vi "1.0.1_Set_SKU_Config.vi"(8 "error in (no error)":errorcluster, 10 "?":T1, 11 "Message Queue out":T2) -> (0 "error out":errorcluster, 1 "Flow":string, 2 "Data":T1, 3 "Message Queue Out":T2)   [LabVIEW 2017]
uses:
  DIPC 692 Daemon API/typdef/destination.ctl
  Depends/AMC/subVIs/TypeDefs/amc_Message Queue.ctl
  Depends/AMC/subVIs/TypeDefs/amc_Message.ctl
  Depends/Tools/Keyed Array/Tools_KeyedArray KeyedArray.ctl
  Ctrls/Data.ctl
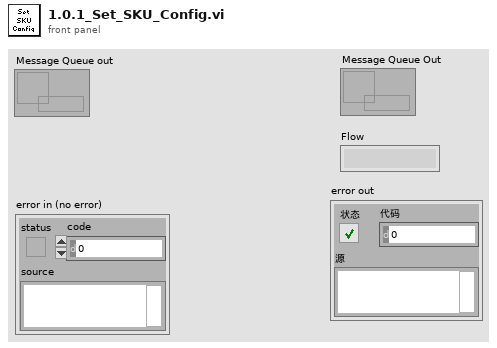
[diagram p1: front panel]
types:
  T1 = typedef "Data.ctl" = cluster{"SN":string, "Start Time":timestamp, "Step Time":timestamp, "Count":cluster{"Total":i32, "OK":i32, "NG":i32, "Yield":dbl}, "Table":string[][], "daemon reference":refnum<k5>, "CT":dbl, "Config":string[][], "Initialisation":cluster{"Set_SKU_Config_With_LMT":string, "FCT_timestamp":string, "sw_version_before":string, "hardware_serial":string, "Backup_DDM_NVM":string, "Flash_SW_follow_SKU":string, "sw_version_after":string, "Set_SKU_Config_base_on_variant":string, "UUT_Ready_Status":string, "Set_DDM_to_EOL_Mode":string, "DDM_Parameter":dbl[], "DDM_Parameter_status":bool[], "Get_Tester_Parameter":dbl[], "Get_Tester_Parameter_status":bool[], "Cal_Tester_Parameter":dbl[], "Cal_Tester_Parameter_status":bool[], "sw_version_before_status":bool, "sw_version_after_status":bool, "Reflashing_Flash_SW_follow_SKU":string, "Set_SKU_Config_With_LMT_status":bool, "FCT_timestamp_status":bool}, "BEMF_Calibration":cluster{"Read_ambient_temperature":dbl, "Set_ambient_temperature_to_DDM":string, "Save_Calibration":string, "Calibration_Vaule":dbl[], "Calibration_Start_Calibration":string, "Calibration_Vaule _B":dbl[], "Calibration_Vaule_status":bool[], "Calibration_Vaule_B_status":bool[]}, "ECO":cluster{"Reset_Power_tune_vaule_to_zero":string, "ECO_Motor_On_with_power_mode":string, "DDM_Parameter":dbl[], "DDM_Parameter_status":bool[], "Get_Tester_Parameter":dbl[], "Get_Tester_Parameter_status":bool[], "Cal_Tester_Parameter":dbl[], "Cal_Tester_Parameter_status":bool[], "DDM_Parameter_after_power_tune":dbl[], "Get_Tester_Parameter_after_power_tune":dbl[], "Cal_Tester_Parameter_after_power_tune":dbl[], "Cal_Tester_Parameter_after_power_tune_status":bool[], "Delta_P":dbl, "ECO_Power_Tune_Set_Delta_Power_tune_value_to_DDM":string, "ECO_Power_Tune_Motor_On_with_power_mode":string, "Reset_BEMF_FISF_calibration":string}, "BOOST":cluster{"DDM_Parameter":dbl[], "DDM_Parameter_status":bool[], "Get_Tester_Parameter":dbl[], "Get_Tester_Parameter_status":bool[], "Cal_Tester_Parameter":dbl[], "Cal_Tester_Parameter_status":bool[], "DDM_Parameter_after_power_tune":dbl[], "Get_Tester_Parameter_after_power_tune":dbl[], "Cal_Tester_Parameter_after_power_tune":dbl[], "Cal_Tester_Parameter_after_power_tune_status":bool[], "airwatts_am_off":dbl, "AW_Delta_(AM_on_and_off)":dbl, "AW_Delta_(AM_on_and_off)_Status":bool, "Delta_P":dbl, "BOOST_Motor_On_with_power_mode":string, "BOOST_Air_Muscle_Check_Turn_off_air_muscle":string, "BOOST_Power_Tune_Set_Delta_Power_tune_value_to_DDM":string, "BOOST_Power_Tune_Motor_On_with_power_mode":string, "BOOST_Stop_motor":string, "BOOST_Save_Calibration":string, "BOOST_Get_AW_Calibration_value":string}, "MAX":cluster{"Max_Motor_On_with_power_mode":string, "Average_Tmag_Data":cluster{"LSI Delta in degC":dbl, "FISF Delta in degc":dbl, "LSI Tmag in degC":dbl, "Fisf Tmag in degC":dbl, "IIR Tmag in degC":dbl}, "DDM_Parameter":dbl[], "DDM_Parameter_status":bool[], "Get_Tester_Parameter":dbl[], "Get_Tester_Parameter_status":bool[], "Cal_Tester_Parameter":dbl[], "BEMF_Finetune":cluster{"eol_bemf_mp_cold_coef_c":dbl, "eol_cold_bemf_fisf_offset":dbl}, "AW_Tune":cluster{"delta_P1":dbl, "delta_P_Setting":dbl}, "DDM_Parameter_after_Airwatts_Tune":dbl[], "Get_Tester_Parameter_after_Airwatts_Tune":dbl[], "Cal_Tester_Parameter_after_Airwatts_Tune":dbl[], "AW_after_Airwatts_Tune":bool, "DDM_Parameter_after_Airwatts_Finetune":dbl[], "Get_Tester_Parameter_after_Airwatts_Finetune":dbl[], "Cal_Tester_Parameter_after_Airwatts_Finetune":dbl[], "AW_after_Airwatts_Finetune":bool, "AW_Finetune":cluster{"delta_P2":dbl, "delta_P_Setting":dbl}, "Delta_Tmag_after_tune":cluster{"LSI Delta in degC":dbl, "FISF Delta in degc":dbl, "LSI Tmag in degC":dbl, "Fisf Tmag in degC":dbl, "IIR Tmag in degC":dbl}, "Hot Bemf in mV":dbl, "DDM_Pressure":dbl, "Delta_Pressure":dbl, " Cold Bemf in mV":dbl, " delta Bemf":dbl, " delta p":dbl, "Delta_Pressure_status":bool, " delta Bemf_status":bool, "LSI Delta in degC_status":bool, "FISF Delta in degc_status":bool, "Motor_On_with_power_mode_after_Airwatts_Tune":string, "Airwatts_Finetune_Motor_On_with_power_mode":string, "Airwatts_Finetune_Stop_motor":string, "Max_check_derate_status":string, "Max_Stop_motor":string, "Max_Save_Calibration":string, "AW":bool, "Max_check_derate_status_status":bool, "Average_All_data":dbl[][], "Average_Tmag_Data_status":bool[], "Average_Tmag_Data_after_tune_status":bool[]}, "Task_Detect_Calib":cluster{"LL":cluster{"DDM_Parameter":dbl[], "DDM_Parameter_status":bool[], "Get_Tester_Parameter":dbl[], "Get_Tester_Parameter_status":bool[], "Set_task_detect_A":dbl, "LL_Motor_On":string}, "HL":cluster{"DDM_Parameter":dbl[], "DDM_Parameter_status":bool[], "Get_Tester_Parameter":dbl[], "Get_Tester_Parameter_status":bool[], "Set_task_detect_B":dbl, "HL_Motor_On":string, "HL_Motor_Stop":string}, "LH":cluster{"DDM_Parameter":dbl[], "DDM_Parameter_status":bool[], "Get_Tester_Parameter":dbl[], "Get_Tester_Parameter_status":bool[], "Set_task_detect_C":dbl, "LH_Motor_On":string}, "HH":cluster{"DDM_Parameter":dbl[], "DDM_Parameter_status":bool[], "Get_Tester_Parameter":dbl[], "Get_Tester_Parameter_status":bool[], "Set_task_detect_D":dbl, "HH_Motor_On":string, "HH_Set_calibration_eol_inlet_blockage":string, "HH_Motor_Stop":string, "HH_Save_calibration":string}, "Get_eol_inlet_blockage_E":dbl, "Calib_vaule":cluster{"Get_task_detect_LL":dbl, "Get_task_detect_HL":dbl, "Get_task_detect_LH":dbl, "Get_task_detect_HH":dbl, "eol_inlet_blockage":dbl}, "Reset_all_task_detect_calibration_parameter":string, "calibrated temp":dbl, "Set ambient temperature to DDM":string, "Set ambient temperature to DDM after task detect":string, "Inlet_Blockage_Calibration":cluster{"DDM_Parameter":dbl[], "DDM_Parameter_status":bool[], "Get_Tester_Parameter":dbl[], "Get_Tester_Parameter_status":bool[], "Inlet_Blockage_Calibration_Motor_On":string, "Calibrate Inlet Blockage":string}}, "good":cluster{"Write_Product_TS":cluster{"TIMESTAMP":i64, "RIG_ID":i64, "PASSMARK_ID":i64, "PASSMARK_REV":i64}, "Read_Product_TS":cluster{"TIMESTAMP":i64, "RIG_ID":i64, "PASSMARK_ID":i64, "PASSMARK_REV":i64}, "Good_Clear_NVM_Error":string, "Good_Set_DDM_to_Product_mode":string, "Good_Write_Product_Timestamp":string, "Good_Read_Product_Timestamp":string, "Good_Backup_DDM_NVM":string, "Good_Set_Secuity_Bit":string, "Good_Set_Calibration_Lock":string, "Good_Check_Secuity_Bit":string, "Good_Check_Secuity_Bit_Stauts":bool}, "Buyoff":cluster{"bit_status":string, "cold_bemf_temp":dbl, "BEMF_Calib_data":dbl[], "AW_Tune_Calib_data":dbl[], "task_Calib_data":dbl[], "Read_Product_TS":cluster{"TIMESTAMP":i64, "RIG_ID":i64, "PASSMARK_ID":i64, "PASSMARK_REV":i64}, "lock_status":string, "Functionality_Buyoff_Get_Product_Timestamp":string}, "UUT_Type":enum16{"692", "692B", "692D"}, "NG":cluster{"NG_Read_Error":string, "NG_Change_to_FCT_mode":string, "NG_Backup_DDM_NVM":string}, "OK/NG":bool}
  T2 = typedef "amc_Message Queue.ctl" = refnum<queue>
  T3 = typedef "HD Config.ctl" = cluster{" PC":cluster{"PC Address":u8[], "PC Port":i32}, "FCO":cluster{"COM":refnum<visa-resource-name>, "Baudrate":u32}, "DC Power ":cluster{"COM":refnum<visa-resource-name>, "Baudrate":u32}, "PW3336":cluster{"COM":refnum<visa-resource-name>, "Baudrate":u32}, "Lefoo":cluster{"COM":refnum<visa-resource-name>, "Baudrate":u32}, "AI Model":cluster{"COM":refnum<visa-resource-name>, "Baudrate":u32}, "DIPC":cluster{"COM":refnum<visa-resource-name>}, "Daemon":cluster{"IP Address":string, "Port":u16}, "Motor":cluster{"COM":refnum<visa-resource-name>, "Baudrate":u32}}
  T4 = typedef "destination.ctl" = string
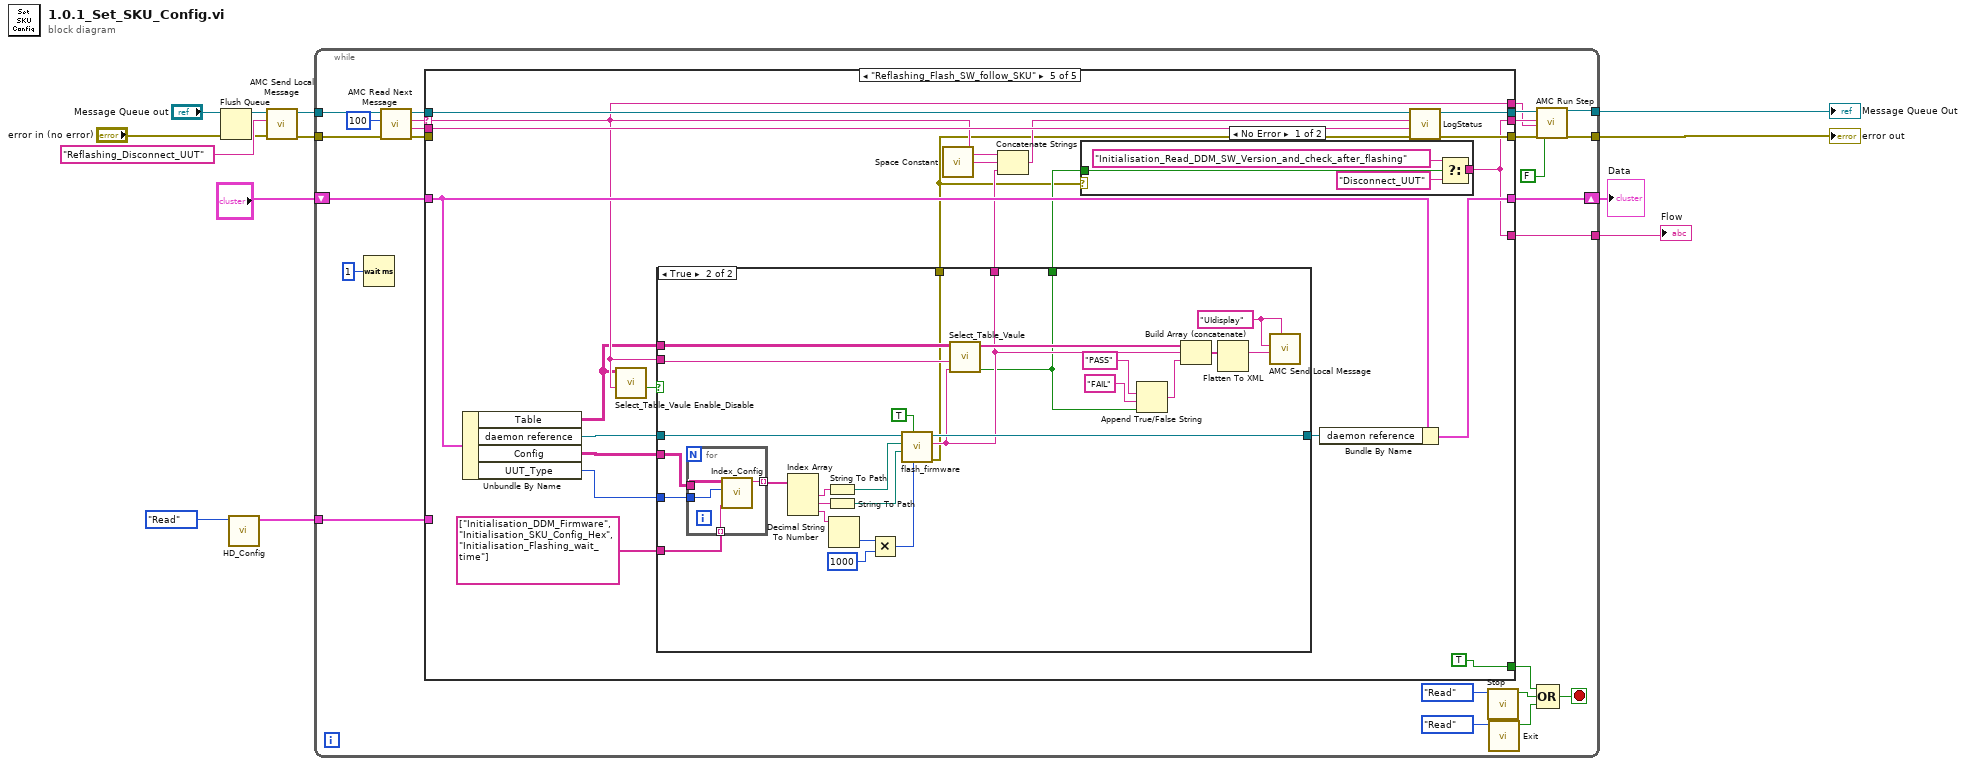
[diagram p0: block diagram]
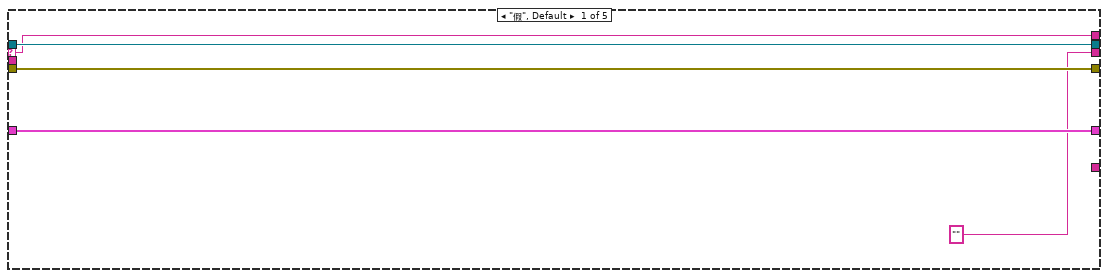
[diagram p2: hidden frame]
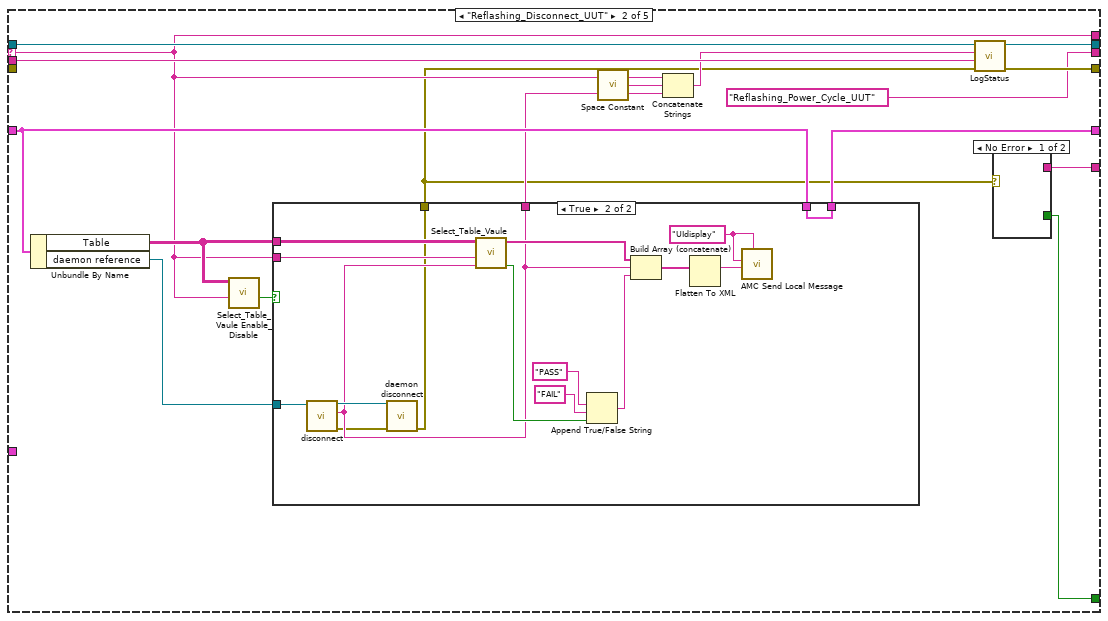
[diagram p3: hidden frame]
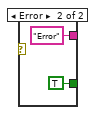
[diagram p4: hidden frame]
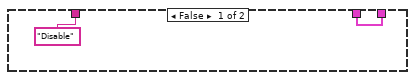
[diagram p5: hidden frame]
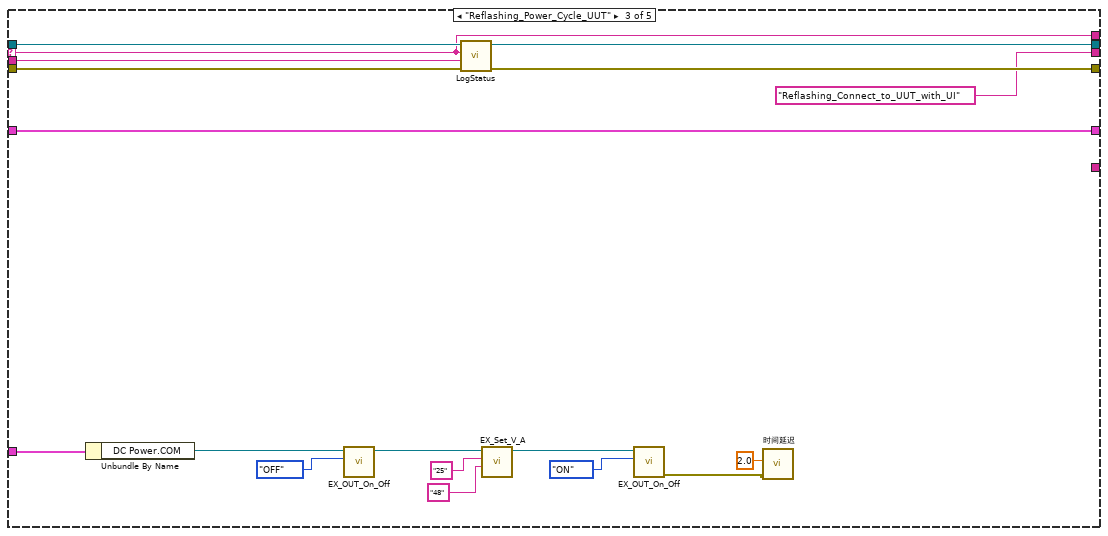
[diagram p6: hidden frame]
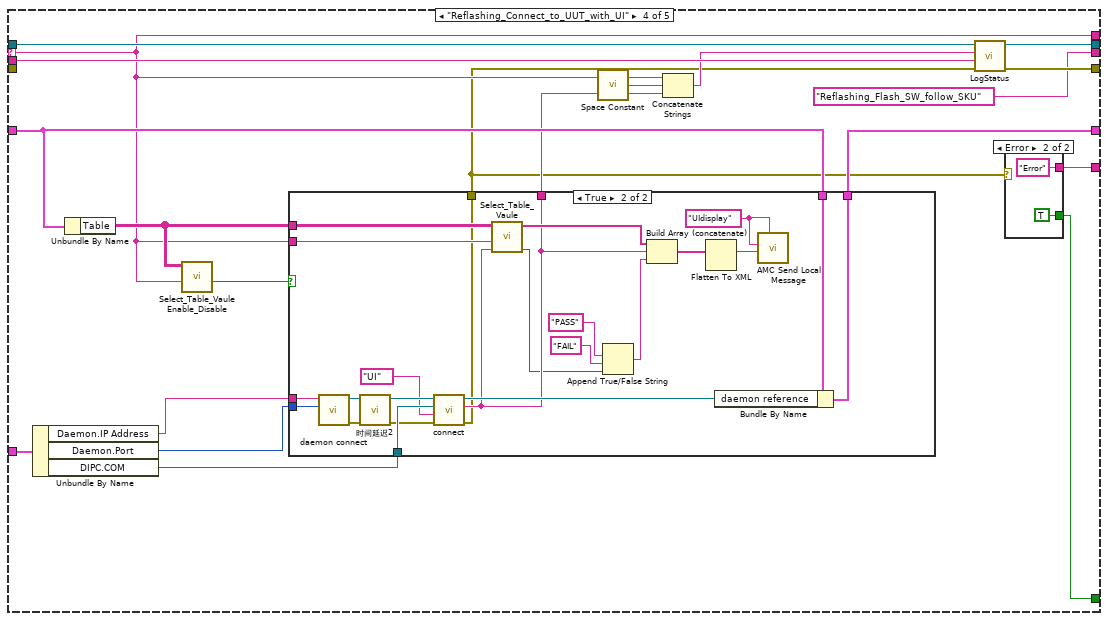
[diagram p7: hidden frame]
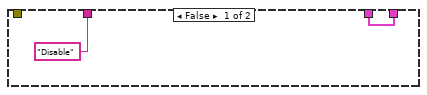
[diagram p9: hidden frame]
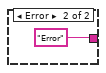
[diagram p10: hidden frame]
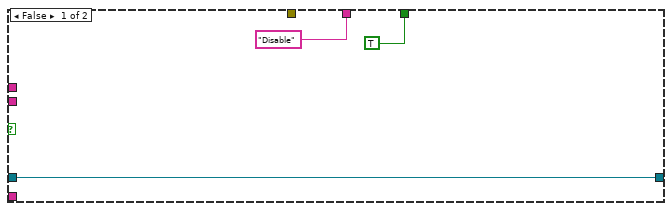
[diagram p11: hidden frame]
diagram:
  n1 = Flush Queue(queue="Message Queue out") -> (queue out=w3:T2)  [unwired: 1 in, 2 out]
  n2 = call "HD_Config.vi"("Step"=enum16{"Initial", "Write", "Read"}."Read") -> ("HD Config out"=w5:T3)  [unwired: 9 in, 1 out]
  n3 = call "AMC Send Local Message.vi"("error in (no error)"="error in (no error)", "Message Name"="Reflashing_Disconnect_UUT", "Message Queue in"=w3) -> ("error out"=w10:errorcluster, "Message Queue out"=w11:T2)  [unwired: 7 in]
  n4 = while {
    tunnel: w11 -> [w38]
    tunnel: [w34] -> w2
    tunnel: w10 -> [w32]
    tunnel: [w29] -> w1
    shift-right: [w25] -> w7
    shift-left: "?" -> [w26]
    tunnel: w5 -> [w24]
    tunnel: [w20] -> w4
    stop <- w14 stop-if-true
    n5 = Wait (ms)(milliseconds to wait=u32 1 ("等待时间（毫秒）")) -> ()  [unwired: 1 out]
    n6 = call "AMC Read Next Message.vi"("error in (no error)"=w32, "timeout (1ms)"=100, "Message Queue in"=w38) -> ("error out"=w31:errorcluster, "Message Value"=w22:string, "Message Name"=w36:string, "Message Queue out"=w37:T2)  [unwired: 1 in, 4 out]
    n7 = case shown="\"Reflashing_Flash_SW_follow_SKU\"" w36 {
      selector: w36 -> [w40 w49 w91 w102 w151]
      tunnel: w37 -> [w43 w59 w96 w115 w161]
      tunnel: [w43 w59 w96 w115 w161] -> w35
      tunnel: w31 -> [w42 _ w94 _ _]
      tunnel: [w42 w58 w93 w114 w160] -> w30
      tunnel: [_ w45 _ w98 TRUE] -> w15
      tunnel: w26 -> [w41 w54 w95 w107 w157]
      tunnel: [w41 w55 w95 w108 w156] -> w25
      tunnel: w22 -> [_ w57 w92 w113 w159]
      tunnel: [w40 w49 w91 w102 w151] -> w21
      tunnel: w24 -> [_ _ w85 w111 _]
      tunnel: ["" "Reflashing_Power_Cycle_UUT" "Reflashing_Connect_to_UUT_with_UI" "Reflashing_Flash_SW_follow_SKU" w145] -> w23
      tunnel: [_ w46 _ w99 w145] -> w20
      frame "假", Default {
      }
      frame "Reflashing_Disconnect_UUT" {
        n8 = Unbundle By Name(w54) -> ("Table"=w50:string[][], "daemon reference"=w47:refnum<k5>)
        n9 = call "Select_Table_Vaule Enable_Disable.vi"("Action"=w49, "Table"=w50) -> ("Enable"=w48:bool)  [unwired: 8 in, 1 out]
        n10 = case shown="True" w48 {
          tunnel: [w63 w66] -> w55
          tunnel: w54 -> [w63 w66]
          tunnel: ["Disable" ("response") w67] -> w51
          tunnel: w50 -> [_ w71]
          tunnel: w49 -> [_ w70]
          tunnel: w47 -> [_ w68]
          tunnel: [_ w64] -> w44
          frame False {
          }
          frame True {
            w78 = "UIdisplay" ("Process (\"\" - local)")
            n11 = call "disconnect.vi"("daemon reference in"=w68) -> ("error out"=w65:errorcluster, "response"=w67:string, "daemon reference out"=w69:refnum<k5>)  [unwired: 7 in, 1 out]
            n12 = call "daemon disconnect.vi"("error in (no error)"=w65, "daemon reference in"=w69) -> ("error out"=w64:errorcluster)  [unwired: 9 in]
            n13 = call "Select_Table_Vaule.vi"("Vaule"=w67, "Action"=w70, "Table"=w71) -> ("Result"=w72:bool, "vaule"=w79:string[])  [unwired: 7 in]
            n14 = Append True/False String(1:w72, 2:"FAIL" ("真字符串"), 3:"PASS" ("真字符串")) -> (0:w73:string)  [unwired: 1 in]
            n15 = Build Array (concatenate)(w79, w67, w73) -> (w77:string[])
            n16 = Flatten To XML(anything=w77) -> (xml string=w76:string)
            n17 = call "AMC Send Local Message.vi"("Process (\"\" - local)"=w78, "Message Value"=w76, "Message Name"=w78) -> ()  [unwired: 7 in, 2 out]
          }
        }
        n18 = call <vilib>:"Space Constant.vi"() -> ("String"=w52:string)
        n19 = Concatenate Strings(w49, w52, w51) -> (w53:string)
        n20 = call "LogStatus.vi"("error in (no error)"=w44, "last message"=w57, "message"=w53) -> ("error  out"=w58:errorcluster)  [unwired: 8 in]
        n21 = case shown="No Error" w44 {
          tunnel: [_ TRUE] -> w45
          tunnel: [_ "Error"] -> w46
          frame No Error {
          }
          frame Error {
          }
        }
      }
      frame "Reflashing_Power_Cycle_UUT" {
        n22 = Unbundle By Name(w85) -> ("DC Power.COM"=w83:refnum<visa-resource-name>)
        n23 = call "EX_OUT_On_Off.vi"("Mode"=enum16{"ON", "OFF"}."OFF", "VISA resource name"=w83) -> ("VISA资源名称输出"=w82:refnum<visa-resource-name>)  [unwired: 8 in, 1 out]
        n24 = call "LogStatus.vi"("error in (no error)"=w94, "last message"=w92, "message"=w91) -> ("error  out"=w93:errorcluster)  [unwired: 8 in]
        n25 = call "EX_Set_V_A.vi"("current"="48", "voltage"="25", "VISA resource name"=w82) -> ("VISA资源名称输出"=w87:refnum<visa-resource-name>)  [unwired: 7 in, 1 out]
        n26 = call "EX_OUT_On_Off.vi"("Mode"=enum16{"ON", "OFF"}."ON", "VISA resource name"=w87) -> ("error out"=w81:errorcluster)  [unwired: 8 in, 1 out]
        n27 = call "时间延迟"("error in (no error)"=w81, "Delay Time (s)"=2.0) -> ()  [unwired: 9 in, 1 out]
      }
      frame "Reflashing_Connect_to_UUT_with_UI" {
        n28 = Unbundle By Name(w111) -> ("Daemon.IP Address"=w100:string, "Daemon.Port"=w110:u16, "DIPC.COM"=w109:refnum<visa-resource-name>)
        n29 = Unbundle By Name(w107) -> ("Table"=w103:string[][])
        n30 = call "Select_Table_Vaule Enable_Disable.vi"("Action"=w102, "Table"=w103) -> ("Enable"=w101:bool)  [unwired: 8 in, 1 out]
        n31 = case shown="True" w101 {
          tunnel: w110 -> [_ w141]
          tunnel: w109 -> [_ w140]
          tunnel: [w119 w139] -> w108
          tunnel: w107 -> [w119 w138]
          tunnel: w100 -> [_ w133]
          tunnel: ["Disable" ("response") w125] -> w104
          tunnel: w103 -> [_ w123]
          tunnel: w102 -> [_ w122]
          tunnel: [_ w120] -> w97
          frame False {
          }
          frame True {
            w131 = "UIdisplay" ("Process (\"\" - local)")
            n32 = call "daemon connect.vi"("port (6543)"=w141, "address (localhost)"=w133) -> ("error out"=w135:errorcluster, "daemon reference out"=w136:refnum<k5>)  [unwired: 8 in]
            n33 = call "时间延迟2"("error in (no error)"=w135) -> ("error out"=w134:errorcluster)  [unwired: 10 in]
            n34 = call "connect.vi"("error in (no error)"=w134, "Target"=T4 "UI", "physical connection"=w140, "daemon reference in"=w136) -> ("error out"=w120:errorcluster, "response"=w125:string, "daemon reference out"=w132:refnum<k5>)  [unwired: 3 in, 2 out]
            n35 = call "Select_Table_Vaule.vi"("Vaule"=w125, "Action"=w122, "Table"=w123) -> ("Result"=w124:bool, "vaule"=w137:string[])  [unwired: 7 in]
            n36 = Append True/False String(1:w124, 2:"FAIL" ("真字符串"), 3:"PASS" ("真字符串")) -> (0:w126:string)  [unwired: 1 in]
            n37 = Build Array (concatenate)(w137, w125, w126) -> (w130:string[])
            n38 = Flatten To XML(anything=w130) -> (xml string=w129:string)
            n39 = Bundle By Name(cluster=w138, "daemon reference"=w132) -> (w139:T1)
            n40 = call "AMC Send Local Message.vi"("Process (\"\" - local)"=w131, "Message Value"=w129, "Message Name"=w131) -> ()  [unwired: 7 in, 2 out]
          }
        }
        n41 = call <vilib>:"Space Constant.vi"() -> ("String"=w105:string)
        n42 = Concatenate Strings(w102, w105, w104) -> (w106:string)
        n43 = call "LogStatus.vi"("error in (no error)"=w97, "last message"=w113, "message"=w106) -> ("error  out"=w114:errorcluster)  [unwired: 8 in]
        n44 = case shown="Error" w97 {
          tunnel: [_ TRUE] -> w98
          tunnel: [_ "Error"] -> w99
          frame No Error {
          }
          frame Error {
          }
        }
      }
      frame "Reflashing_Flash_SW_follow_SKU" {
        n45 = Unbundle By Name(w157) -> ("Table"=w150:string[][], "daemon reference"=w158:refnum<k5>, "Config"=w148:string[][], "UUT_Type"=w144:enum16{"692", "692B", "692D"})
        n46 = call "Select_Table_Vaule Enable_Disable.vi"("Action"=w151, "Table"=w150) -> ("Enable"=w149:bool)  [unwired: 8 in, 1 out]
        n47 = case shown="True" w149 {
          tunnel: w158 -> [w169 w190]
          tunnel: [w169 w189] -> w155
          tunnel: ["Disable" ("software string") w185] -> w152
          tunnel: w151 -> [_ w188]
          tunnel: w150 -> [_ w187]
          tunnel: w148 -> [_ w173]
          tunnel: [TRUE w183] -> w146
          tunnel: w144 -> [_ w172]
          tunnel: string[] ["Initialisation_DDM_Firmware", "Initialisation_SKU_Config_Hex", "Initialisation_Flashing_wait_time"] -> [_ w171]
          tunnel: [_ w170] -> w142
          frame False {
          }
          frame True {
            w196 = "UIdisplay" ("Process (\"\" - local)")
            n48 = for {
              tunnel: w173 -> [w200]
              tunnel: w172 -> [w199]
              tunnel: w171 -> [w198] mode=indexing
              tunnel: [w197] -> w178 mode=indexing
              n49 = call "Index_Config.vi"("Action"=w198, "UUT_Type"=w199, "config"=w200) -> ("data"=w197:string)  [unwired: 8 in]
            }
            n50 = Index Array(array=w178) -> (element #1=w179:string, element #2=w180:string, element #3=w181:string)  [unwired: 3 in]
            n51 = String To Path(string=w179) -> (path=w176:path)
            n52 = String To Path(string=w180) -> (path=w175:path)
            n53 = Decimal String To Number(string=w181) -> (number=w182:i32)  [unwired: 2 in, 1 out]
            n54 = Multiply(x=w182, y=1000) -> (x*y=w174:i32)
            n55 = call "flash_firmware.vi"("timeout (25000ms)"=w174, "SW 4.1 and above?"=TRUE, "SIV bin path"=w175, "firmware path"=w176, "daemon reference in"=w190) -> ("error out"=w170:errorcluster, "response"=w185:string, "daemon reference out"=w189:refnum<k5>)  [unwired: 3 in, 1 out]
            n56 = call "Select_Table_Vaule.vi"("Vaule"=w185, "Action"=w188, "Table"=w187) -> ("Result"=w183:bool, "vaule"=w186:string[])  [unwired: 7 in]
            n57 = Append True/False String(1:w183, 2:"FAIL" ("真字符串"), 3:"PASS" ("真字符串")) -> (0:w191:string)  [unwired: 1 in]
            n58 = Build Array (concatenate)(w186, w185, w191) -> (w195:string[])
            n59 = Flatten To XML(anything=w195) -> (xml string=w194:string)
            n60 = call "AMC Send Local Message.vi"("Process (\"\" - local)"=w196, "Message Value"=w194, "Message Name"=w196) -> ()  [unwired: 7 in, 2 out]
          }
        }
        n61 = call <vilib>:"Space Constant.vi"() -> ("String"=w154:string)
        n62 = Concatenate Strings(w151, w154, w152) -> (w153:string)
        n63 = case shown="No Error" w142 {
          tunnel: w146 -> [w165 _]
          tunnel: [w162 "Error"] -> w145
          frame No Error {
            n64 = Select(t="Initialisation_Read_DDM_SW_Version_and_check_after_flashing", s=w165, f="Disconnect_UUT") -> (s? t:f=w162:string)
          }
          frame Error {
          }
        }
        n65 = Bundle By Name(cluster=w157, "daemon reference"=w155) -> (w156:T1)
        n66 = call "LogStatus.vi"("error in (no error)"=w142, "last message"=w159, "message"=w153) -> ("error  out"=w160:errorcluster)  [unwired: 8 in]
      }
    }
    n67 = call "Stop.vi"("Step"=enum16{"Initial", "Write", "Read"}."Read") -> ("Stop Out"=w17:bool)  [unwired: 9 in, 1 out]
    n68 = call "Exit.vi"("Step"=enum16{"Initial", "Write", "Read"}."Read" ("step")) -> ("Exit Out"=w16:bool)  [unwired: 9 in, 1 out]
    n69 = call "AMC Run Step.vi"("Message Queue In"=w35, "Message Name"=w23, "Message Value"=w21, "error in (no error)"=w30, "Mli/Sig"=FALSE) -> ("Message Queue Out"=w34:T2, "error out"=w29:errorcluster)  [unwired: 13 in]
    n70 = Compound Arithmetic op=OR(w15, w17, w16) -> (w14:bool)
  }
  "Message Queue Out" <- w2
  "error out" <- w1
  "Data" <- w7
  "Flow" <- w4
